vi "TSM Clear DAQmx Tasks And Reset Devices.vi"(0 "TSM context":T1) -> (15 "error out":errorcluster)   [LabVIEW 2019]
doc: "Use this VI to reset and clear all tasks for all NI-DAQmx instruments in the Semiconductor Module Context."
uses:
  <vilib>/NI_TestStand_SemiconductorModule/NI_TestStand_Semiconductor_Module.lvlibp/PinMap/General/SemiconductorModuleContext.ctl
  <resource>/objmgr/daqmx.rc
  <vilib>/NI_TestStand_SemiconductorModule/NI_TestStand_Semiconductor_Module.lvlibp
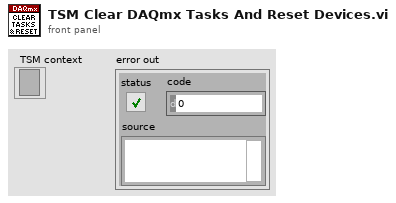
[diagram p1: front panel]
types:
  T1 = typedef "NI_TestStand_Semiconductor_Module.lvlibp/SemiconductorModuleContext.ctl" = refnum<k7>
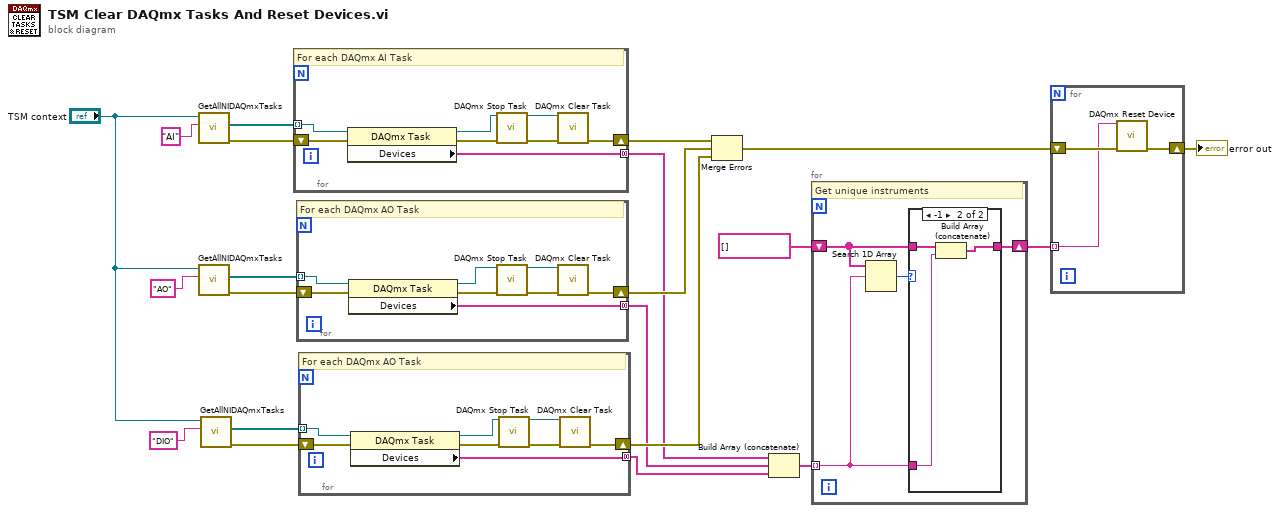
[diagram p0: block diagram]
diagram:
  n1 = call <vilib>:"GetAllNIDAQmxTasks.vi"("Task Type"="AI", "Semiconductor Module Context"="TSM context") -> ("error out"=w20:errorcluster, "DAQmx Tasks"=w11:refnum<k21>[])  [unwired: 7 in, 1 out]
  n2 = call <vilib>:"GetAllNIDAQmxTasks.vi"("Task Type"="AO", "Semiconductor Module Context"="TSM context") -> ("error out"=w17:errorcluster, "DAQmx Tasks"=w10:refnum<k21>[])  [unwired: 7 in, 1 out]
  n3 = call <vilib>:"GetAllNIDAQmxTasks.vi"("Task Type"="DIO", "Semiconductor Module Context"="TSM context") -> ("error out"=w15:errorcluster, "DAQmx Tasks"=w9:refnum<k21>[])  [unwired: 7 in, 1 out]
  n4 = for {
    tunnel: w11 -> [w24] mode=indexing
    shift-right: [w27] -> w21
    shift-left: w20 -> [w29]
    tunnel: [w22] -> w4 mode=concatenating
    # "For each DAQmx AI Task"
    n5 = property class="DAQmx Task"(reference=w24, error in=w29) -> (reference out=w23:refnum<k21>, error out=w25:errorcluster, "Devices"=w22:tag[])
    n6 = call <vilib>:"DAQmx Stop Task.vi"("task/channels in"=w23, "error in"=w25) -> ("task out"=w28:refnum<k21>, "error out"=w26:errorcluster)  [unwired: 12 in]
    n7 = call <vilib>:"DAQmx Clear Task.vi"("task in"=w28, "error in"=w26) -> ("error out"=w27:errorcluster)  [unwired: 13 in]
  }
  n8 = for {
    tunnel: w10 -> [w32] mode=indexing
    shift-right: [w35] -> w16
    shift-left: w17 -> [w37]
    tunnel: [w30] -> w3 mode=concatenating
    # "For each DAQmx AO Task"
    n9 = property class="DAQmx Task"(reference=w32, error in=w37) -> (reference out=w31:refnum<k21>, error out=w33:errorcluster, "Devices"=w30:tag[])
    n10 = call <vilib>:"DAQmx Stop Task.vi"("task/channels in"=w31, "error in"=w33) -> ("task out"=w36:refnum<k21>, "error out"=w34:errorcluster)  [unwired: 12 in]
    n11 = call <vilib>:"DAQmx Clear Task.vi"("task in"=w36, "error in"=w34) -> ("error out"=w35:errorcluster)  [unwired: 13 in]
  }
  n12 = for {
    tunnel: w9 -> [w40] mode=indexing
    shift-right: [w43] -> w12
    shift-left: w15 -> [w45]
    tunnel: [w38] -> w2 mode=concatenating
    # "For each DAQmx AO Task"
    n13 = property class="DAQmx Task"(reference=w40, error in=w45) -> (reference out=w39:refnum<k21>, error out=w41:errorcluster, "Devices"=w38:tag[])
    n14 = call <vilib>:"DAQmx Stop Task.vi"("task/channels in"=w39, "error in"=w41) -> ("task out"=w44:refnum<k21>, "error out"=w42:errorcluster)  [unwired: 12 in]
    n15 = call <vilib>:"DAQmx Clear Task.vi"("task in"=w44, "error in"=w42) -> ("error out"=w43:errorcluster)  [unwired: 13 in]
  }
  n16 = Merge Errors(w21, w16, w12) -> (w5:errorcluster)
  n17 = Build Array (concatenate)(w4, w3, w2) -> (w1:tag[])
  n18 = for {
    shift-right: [w47] -> w7
    shift-left: tag[] [] ("Devices") -> [w48]
    tunnel: w1 -> [w46] mode=indexing
    # "Get unique instruments"
    n19 = Search 1D Array(1D array=w48, element=w46) -> (index of element=w49:i32)  [unwired: 1 in]
    n20 = case shown="-1" w49 {
      tunnel: w48 -> [w50 w53]
      tunnel: [w50 w52] -> w47
      tunnel: w46 -> [_ w51]
      frame Default {
      }
      frame -1 {
        n21 = Build Array (concatenate)(w53, w51) -> (w52:tag[])
      }
    }
  }
  n22 = for {
    shift-right: [w55] -> w6
    shift-left: w5 -> [w56]
    tunnel: w7 -> [w54] mode=indexing
    n23 = call <vilib>:"DAQmx Reset Device.vi"("device in"=w54, "error in"=w56) -> ("error out"=w55:errorcluster)  [unwired: 13 in]
  }
  "error out" <- w6
